vi "Create RC Client.vi"(8 "error in (no error)":errorcluster, 9 "Port":u16, 10 "address":string, 11 "RemoteControl in":refnum<class "RemoteControl.lvclass">) -> (0 "error out":errorcluster, 3 "RemoteControl out":refnum<class "RemoteControl.lvclass">)   [LabVIEW 2020, in "RemoteControl.lvclass"]
uses:
  RemoteControl.lvclass
  C:/Program Files (x86)/National Instruments/LabVIEW 2020/vi.lib/JKI/JKI SMO/SMO/SMO.lvclass
  Typedefs/RC Process Type--Enum.ctl
  RemoteControl.lvclass/RemoteControl.ctl
  <vilib>/JKI/JKI SMO/SMO/SMO.lvclass
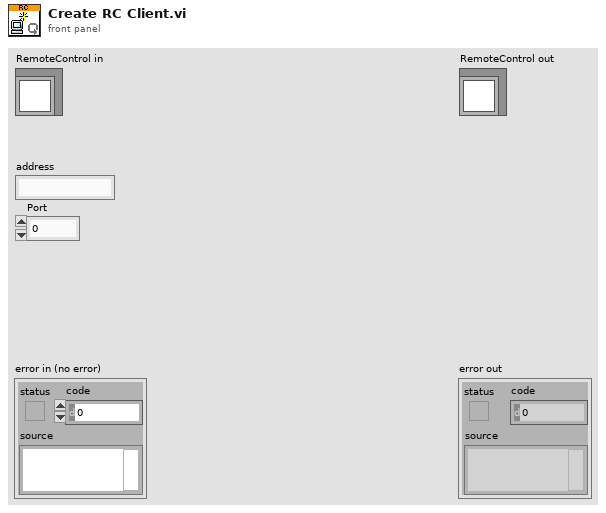
[diagram p1: front panel]
types:
  T1 = typedef "RemoteControl.lvclass/RC Process Type--Enum.ctl" = enum16{"Connection Monitor", "Server", "Client"}
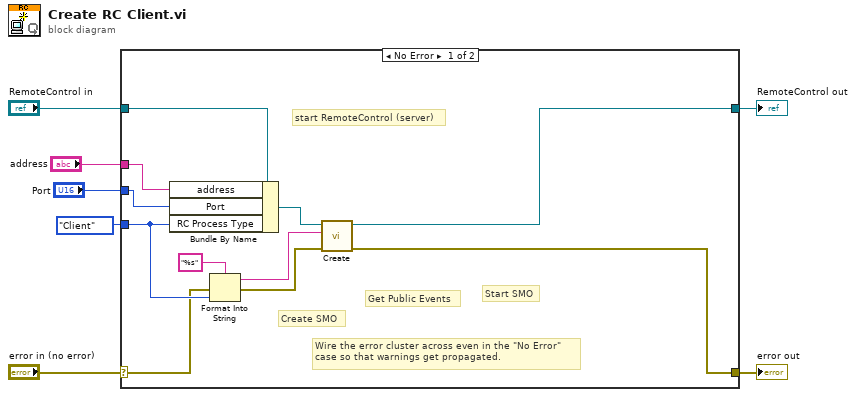
[diagram p0: block diagram]
diagram:
  n1 = case shown="No Error" "error in (no error)" {
    selector: "error in (no error)" -> [w14 w20]
    tunnel: [w11 w20] -> w6
    tunnel: [w10 w19] -> w4
    tunnel: "RemoteControl in" -> [w17 w19]
    tunnel: RC_Process_Type--Enum."Client" ("RC Process Type") -> [w15 _]
    tunnel: "Port" -> [w9 _]
    tunnel: "address" -> [w8 _]
    frame No Error {
      # "start RemoteControl (server)"
      # "Get Public Events"
      # "Start SMO"
      # "Create SMO"
      # "Wire the error cluster across even in the \"No Error\"\ncase so that warnings get propagated."
      n2 = Bundle By Name(cluster=w17, "address"=w8, "Port"=w9, "RC Process Type"=w15) -> (w18:refnum<class "RemoteControl.lvclass">)
      n3 = Format Into String(format string="%s", error in=w14, w15) -> (resulting string=w13:string, error out=w12:errorcluster)  [unwired: 1 in]
      n4 = call <vilib>:"Create.vi"("error in (no error)"=w12, "Subsystem Name (optional)"=w13, "SMO"=w18) -> ("error out"=w11:errorcluster, "SMO out"=w10:refnum<class "RemoteControl.lvclass">)  [unwired: 6 in, 1 out]
    }
    frame Error {
    }
  }
  "error out" <- w6
  "RemoteControl out" <- w4
